vi "XY Graph Add or Replace Plot (by Index).vi"(5 "New Plot Name":string, 6 "Replace Plot (T)?":bool, 7 "Original Plot Name":string, 8 "error in (no error)":errorcluster, 9 "Plot Index":i32, 10 "Plot in":cluster{"X Array":dbl[], "Y Array":dbl[]}, 11 "XYGraph in":T1) -> (0 "error out":errorcluster, 1 "Message":string)   [LabVIEW 2021, in "XY Graph Add-Ons.lvlib"]
uses:
  XY Graph Add-Ons.lvlib
  XY Graph Refnum.ctl
  XY Graph Add Single Plot with Name.vi
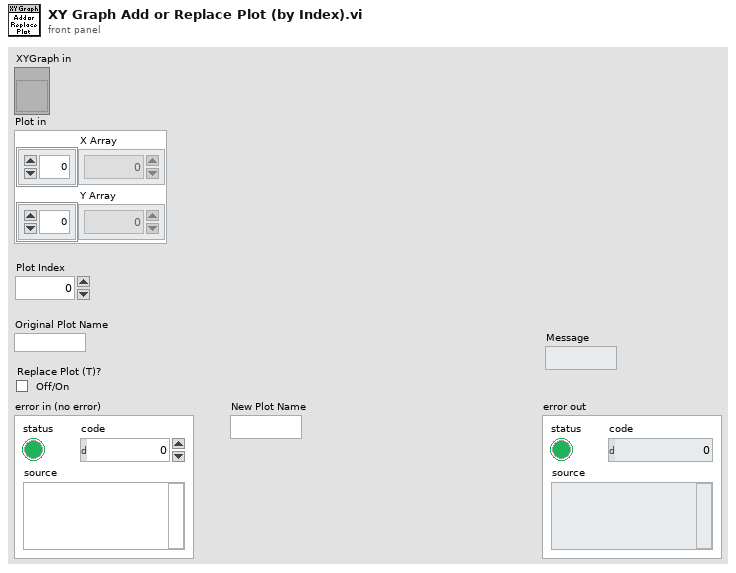
[diagram p1: front panel]
types:
  T1 = typedef "XY Graph Add-Ons.lvlib/XY Graph Refnum.ctl" = refnum<vi>
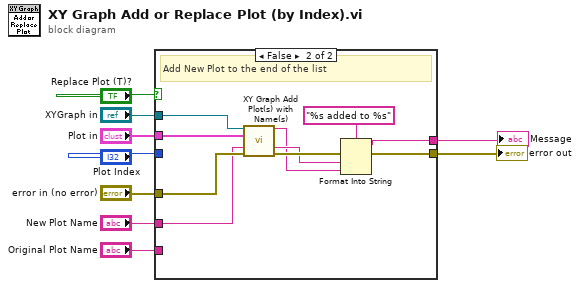
[diagram p0: block diagram]
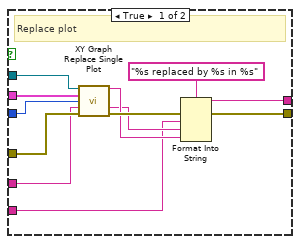
[diagram p2: hidden frame]
diagram:
  n1 = case shown="False" "Replace Plot (T)?" {
    tunnel: "XYGraph in" -> [w15 w31]
    tunnel: [w20 w27] -> w7
    tunnel: [w21 w26] -> w6
    tunnel: "Original Plot Name" -> [w11 _]
    tunnel: "error in (no error)" -> [w18 w30]
    tunnel: "New Plot Name" -> [w17 w22]
    tunnel: "Plot in" -> [w16 w29]
    tunnel: "Plot Index" -> [w10 _]
    frame True {
      # "Replace plot"
      n2 = call "XY Graph Replace Single Plot.vi"("XYGraph Ref in"=w15, "Plot"=w16, "Plot index"=w10, "Plot Name (\"Plot\")"=w17, "error in (no error)"=w18) -> ("XY Graph Caption (or Label)"=w13:string, "Plot Name"=w12:string, "error out"=w14:errorcluster)  [unwired: 7 in, 1 out]
      n3 = Format Into String(format string="%s replaced by %s in %s", error in=w14, w11, w12, w13) -> (resulting string=w21:string, error out=w20:errorcluster)  [unwired: 1 in]
    }
    frame False {
      # "Add New Plot to the end of the list"
      n4 = call-poly "XY Graph Add Plot(s) with Name(s).vi"("XYGraph Ref in"=w31, "Plot"=w29, "Plot Name (\"Plot\")"=w22, "error in (no error)"=w30) -> ("XY Graph Caption (or Label)"=w23:string, "Plot Name"=w24:string, "error out"=w28:errorcluster)  [unwired: 8 in, 1 out]
      n5 = Format Into String(format string="%s added to %s" ("input 1"), error in=w28, w24, w23) -> (resulting string=w26:string, error out=w27:errorcluster)  [unwired: 1 in]
    }
  }
  "error out" <- w7
  "Message" <- w6
